vi "GFITS_GetArrSubSet.vi"(0 "newcom":string, 4 "newkey":string, 5 "stored names":string[](array[string]), 6 "array type":string, 7 "stored vals":T1(array[cluster]), 8 "index":i32, 9 "subset?":bool, 10 "dbs table":string[][](table), 11 "array name":string) -> (2 "arr subset":string[][](array[string]))   [LabVIEW 2016]
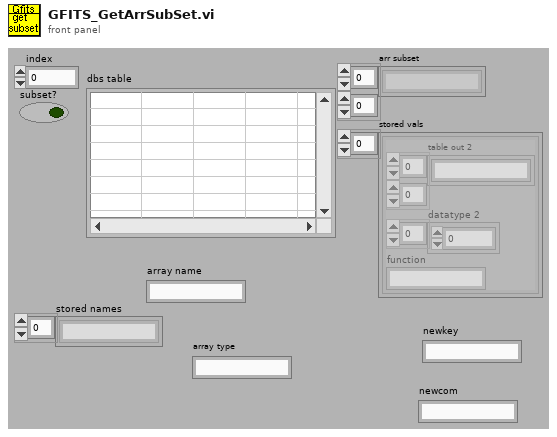
[diagram p1: front panel]
types:
  T1 = cluster{"table out 2":string[][], "datatype 2":u16[], "function":string}[]
  T2 = cluster{"table out 2":string[][], "datatype 2":u16[], "function":string}
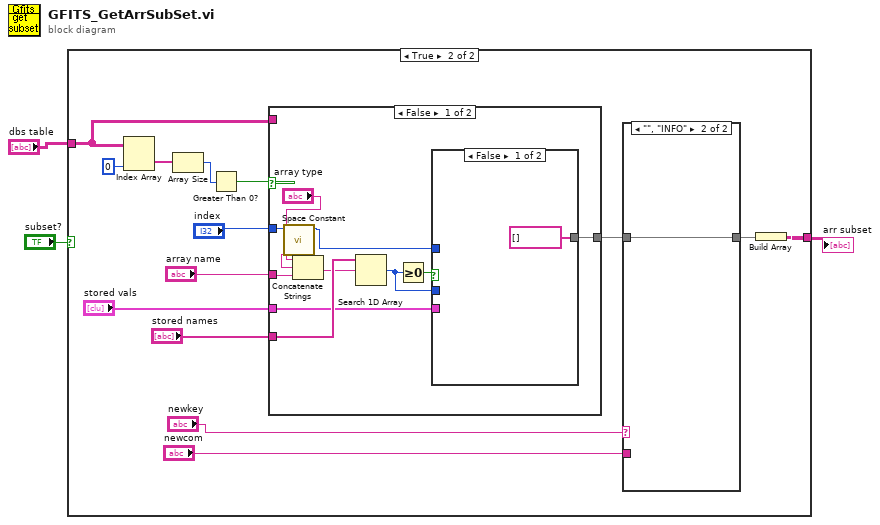
[diagram p0: block diagram]
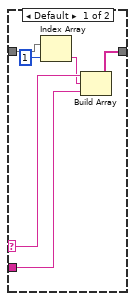
[diagram p3: hidden frame]
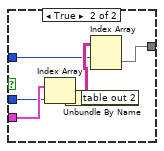
[diagram p4: hidden frame]
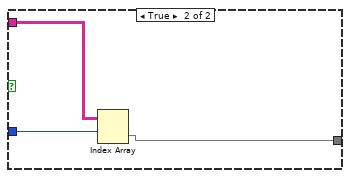
[diagram p5: hidden frame]
diagram:
  n1 = case shown="True" "subset?" {
    tunnel: [w4 w10] -> w3
    tunnel: "dbs table" -> [w4 w9]
    frame False {
    }
    frame True {
      n2 = Index Array(array=w9, index (col)=0 ("disabled index (col)")) -> (element=w17:string[])  [unwired: 1 in]
      n3 = Array Size(array=w17) -> (size(s)=w16:i32)
      n4 = Greater Than 0?(x=w16) -> (x > 0?=w14:bool)
      n5 = case shown="False" w14 {
        tunnel: "index" -> [w31 w45]
        tunnel: w9 -> [_ w44]
        tunnel: "stored vals" -> [w33 _]
        tunnel: "stored names" -> [w35 _]
        tunnel: "array name" -> [w29 _]
        tunnel: [w30 w43] -> w7
        frame False {
          n6 = call <vilib>:"Space Constant.vi"() -> ("String"=w27:string)
          n7 = Concatenate Strings("array type", w27, w29) -> (w26:string)
          n8 = Search 1D Array(1D array=w35, element=w26) -> (index of element=w32:i32)  [unwired: 1 out]
          n9 = Greater Or Equal To 0?(x=w32) -> (x >= 0?=w34:bool)
          n10 = case shown="False" w34 {
            tunnel: w33 -> [_ w42]
            tunnel: w32 -> [_ w41]
            tunnel: w31 -> [_ w38]
            tunnel: [string[] [] ("table out 2") w37] -> w30
            frame False {
            }
            frame True {
              n11 = Index Array(array=w42, index=w41) -> (element=w40:T2)
              n12 = Unbundle By Name(w40) -> ("table out 2"=w39:string[][])
              n13 = Index Array(array=w39, index (row)=w38) -> (element=w37:string[])  [unwired: 1 in]
            }
          }
        }
        frame True {
          n14 = Index Array(array=w44, index (row)=w45) -> (element=w43:string[])  [unwired: 1 in]
        }
      }
      n15 = case shown="\"\", \"INFO\"" "newkey" {
        selector: "newkey" -> [w24 _]
        tunnel: w7 -> [w23 w25]
        tunnel: [w19 w25] -> w6
        tunnel: "newcom" -> [w20 _]
        frame Default {
          n16 = Index Array(array=w23, index=1) -> (element=w21:string)
          n17 = Build Array(w24, w21, w20) -> (w19:string[])
        }
        frame "", "INFO" {
        }
      }
      n18 = Build Array(w6) -> (w10:string[][])
    }
  }
  "arr subset" <- w3
